vi "List_Files.vi"(8 "error in (no error)":errorcluster, 10 "include unused? (T)":bool=TRUE, 11 "Installer in":refnum<class "Installer.lvclass">) -> (0 "error out":errorcluster, 2 "files":T1[](array[typedef]), 3 "Installer out":refnum<class "Installer.lvclass">)   [LabVIEW 2020, in "Installer.lvclass"]
uses:
  <vilib>/AppBuilder/IB_Classes/Installer/Installer.lvclass
  <vilib>/AppBuilder/IB_Classes/Installer/Installer.lvclass/Installer.ctl
  <vilib>/AppBuilder/IB_Classes/Source/File/IB_Source_File.lvclass
  <vilib>/AppBuilder/IB_Classes/Source/IB_Source.lvclass
  <resource>/Framework/Providers/Builds/Installer/CDK_sTypeDef_FileList.ctl
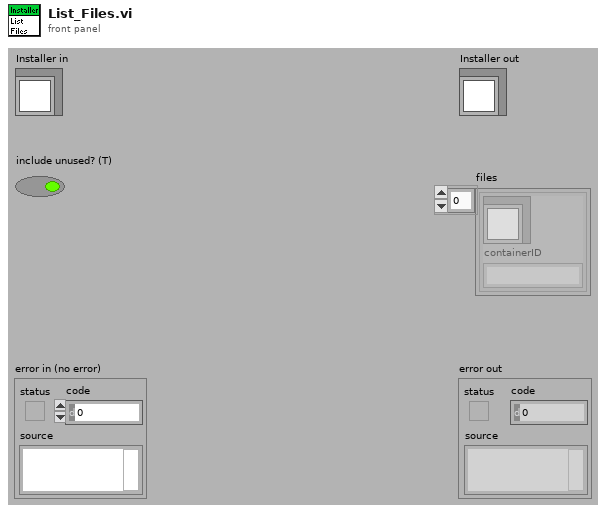
[diagram p1: front panel]
types:
  T1 = typedef "CDK_sTypeDef_FileList.ctl" = cluster{"FileInventory":refnum<class "IB_Source_File.lvclass">, "containerID":string}
  T2 = typedef "IB_Source.ctl" = cluster{"name":string, "sourceTag":string, "destTag":string, "path":path, "eng_installPath":string, "UI_inBuild?":bool, "str ref?":bool}
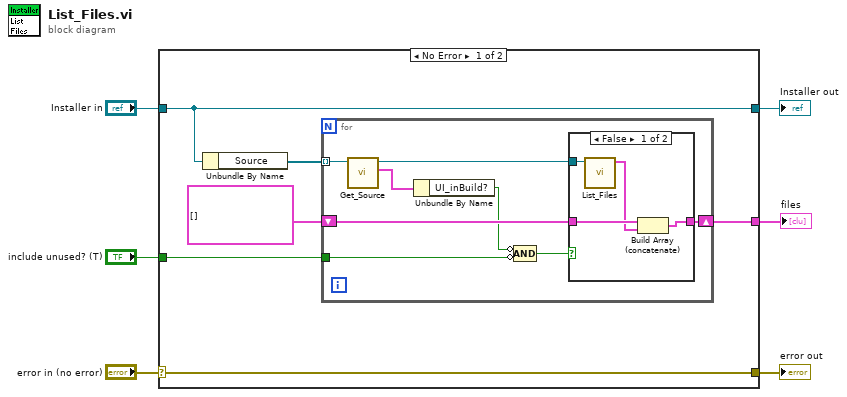
[diagram p0: block diagram]
diagram:
  n1 = case shown="No Error" "error in (no error)" {
    selector: "error in (no error)" -> [w12 w27]
    tunnel: [w12 w27] -> w5
    tunnel: [w11 w26] -> w3
    tunnel: "Installer in" -> [w11 w26]
    tunnel: [w8 _] -> w2
    tunnel: "include unused? (T)" -> [w7 _]
    frame No Error {
      n2 = Unbundle By Name(w11) -> ("Source"=w10:refnum<class "IB_Source.lvclass">[])
      n3 = for {
        tunnel: w10 -> [w18] mode=indexing
        shift-right: [w19] -> w8
        shift-left: T1[] [] ("Files") -> [w20]
        tunnel: w7 -> [w15]
        n4 = call <vilib>:"Get_Source.vi"("IB_Source in"=w18) -> ("data"=w16:T2, "IB_Source out"=w17:refnum<class "IB_Source.lvclass">)  [unwired: 1 in, 8 out]
        n5 = Unbundle By Name(w16) -> ("UI_inBuild?"=w14:bool)
        n6 = Compound Arithmetic op=AND(invert w14, invert w15) -> (w13:bool)
        n7 = case shown="False" w13 {
          tunnel: w20 -> [w24 w25]
          tunnel: [w23 w25] -> w19
          tunnel: w17 -> [w21 _]
          frame False {
            n8 = call-dynamic "List_Files.vi"("IB_Source in"=w21) -> ("Files"=w22:T1[])  [unwired: 1 in, 9 out]
            n9 = Build Array (concatenate)(w24, w22) -> (w23:T1[])
          }
          frame True {
          }
        }
      }
    }
    frame Error {
    }
  }
  "error out" <- w5
  "Installer out" <- w3
  "files" <- w2
